vi "GT Get Gear Event.vi"(0 "cardNum":i16, 1 "pStartPara1":i32, 5 "profile":i16, 7 "pEvent":i16, 9 "pStartPara0":i32, 11 "error in (no error)":errorcluster caption="错误输入（无错误）") -> (3 "pStartPara1 out":i32, 4 "function return":i16, 8 "pEvent out":i16, 10 "pStartPara0 out":i32, 15 "error out":errorcluster caption="错误输出")   [LabVIEW 2020, in "gts.lvlib"]
doc: "GT_API GT_GetGearEvent(short cardNum,short profile,short *pEvent,long *pStartPara0,long *pStartPara1);"
uses:
  gts.lvlib
  dll/32bit/multi_card/gts.dll
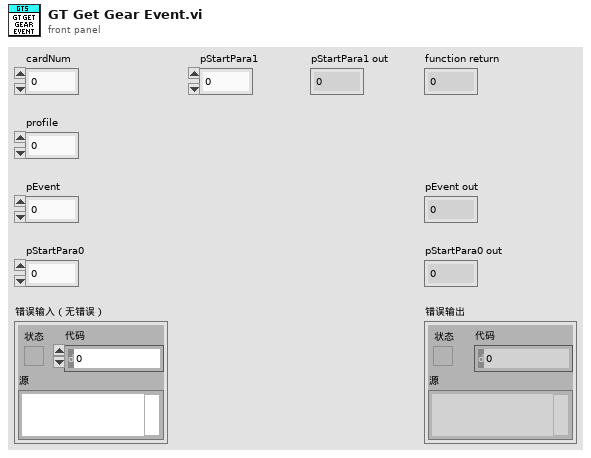
[diagram p1: front panel]
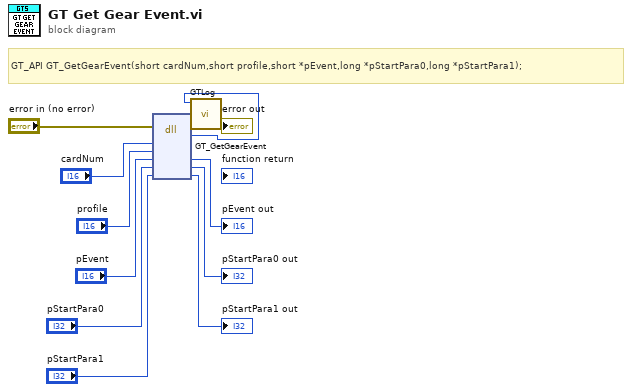
[diagram p0: block diagram]
diagram:
  # "GT_API GT_GetGearEvent(short cardNum,short profile,short *pEvent,long *pStartPara0,long *pStartPara1);"
  n1 = dll-call lib="C:/1228/dll/32bit/multi_card/gts.dll" fn="GT_GetGearEvent"(error in="error in (no error)", "cardNum"="cardNum", "profile"="profile", "pEvent"="pEvent", "pStartPara0"="pStartPara0", "pStartPara1"="pStartPara1") -> (error out=w3:errorcluster, w1:i16, "pEvent"=→"pEvent out":i16, "pStartPara0"=→"pStartPara0 out":i32, "pStartPara1"=→"pStartPara1 out":i32)  [unwired: 4 in, 1 out]
  n2 = call "GTLog.vi"("error in (no error)"=w3, "Numeric"=w1) -> ("error out"=→"error out":errorcluster)  [unwired: 9 in]
